vi "DAQNavi Create Channel(Buffered-CI-Count Value).vi"(0 "task in":i32, 5 "physical channels":string, 11 "error in (no error)":errorcluster) -> (4 "task out":i32, 15 "error out":errorcluster)   [LabVIEW 2020]
uses:
  DAQNavi_LV.dll
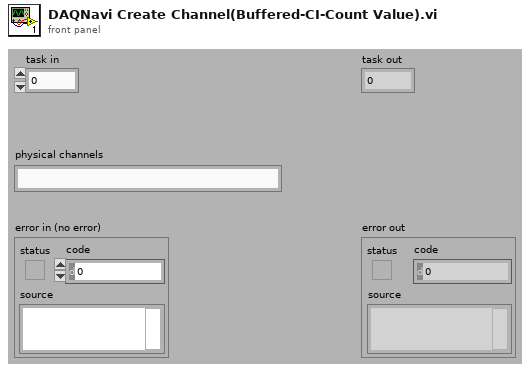
[diagram p1: front panel]
types:
  T1 = enum16{"InstantAI", "OneBufferedAI", "StreamingAI", "StaticAO", "OneWaveformAO", "StreamingAO", "InstantDI", "DIInterrupt", "StaticDO", "EventCounter", "FreqMeter", "OneShot", "TimerPulse", "PwMeter", "PwModulator", "UdCounter", "WaveformAI", "BufferedEventCounter", "BufferedPwMeter", "BufferedPwModulator", "BufferedUdCounter"}
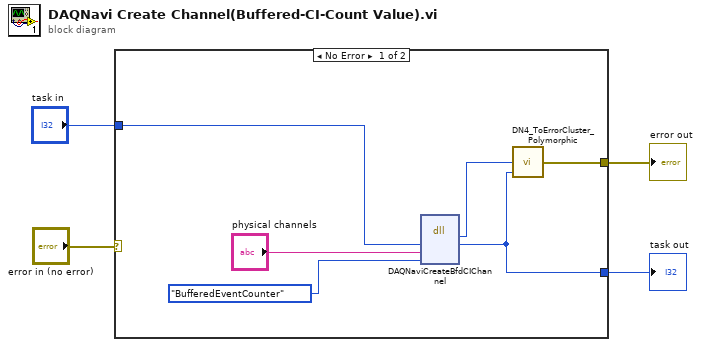
[diagram p0: block diagram]
diagram:
  n1 = case shown="No Error" "error in (no error)" {
    selector: "error in (no error)" -> [_ w11]
    tunnel: "task in" -> [w9 w12]
    tunnel: [w5 w12] -> w2
    tunnel: [w6 w11] -> w1
    frame No Error {
      n2 = dll-call lib="DAQNavi_LV.dll" fn="DAQNaviCreateBfdCIChannel"("taskId"=w9, "physicalChannel"="physical channels", "taskType"=T1."BufferedEventCounter") -> ("return type"=w7:i32, "taskId"=w5:i32)  [unwired: 4 in, 3 out]
      n3 = call "DN4_ToErrorCluster_Polymorphic.vi"("task id"=w5, "error code"=w7) -> ("error out"=w6:errorcluster)  [unwired: 3 out]
    }
    frame Error {
    }
  }
  "task out" <- w2
  "error out" <- w1
